vi "fitImageToWindow.vi"(8 "error in (no error)":errorcluster, 9 "Image Area Size":cluster{"Width":u32, "Height":u32}, 10 "ImageSize":cluster{"x":i32, "y":i32}, 11 "Snapper in":refnum<class "Snapper.lvclass">) -> (0 "error out":errorcluster, 2 "zoomInteger":cluster{dbl, dbl}, 3 "Snapper out":refnum<class "Snapper.lvclass">)   [LabVIEW 2009, in "Views.lvlib" / "Camera.lvlib" / "Snapper.lvclass"]
uses:
  Snapper.lvclass
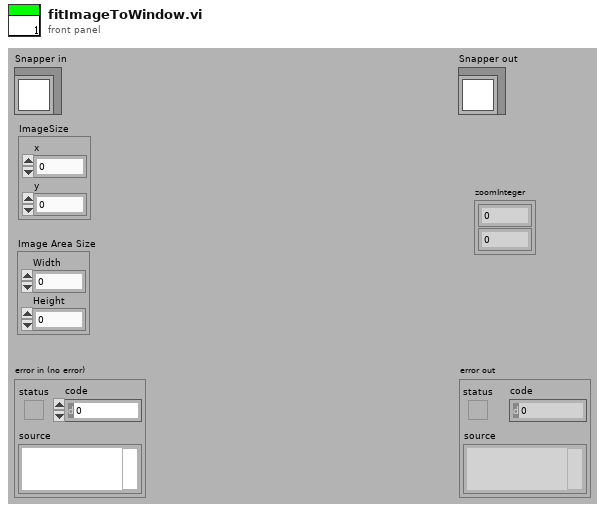
[diagram p1: front panel]
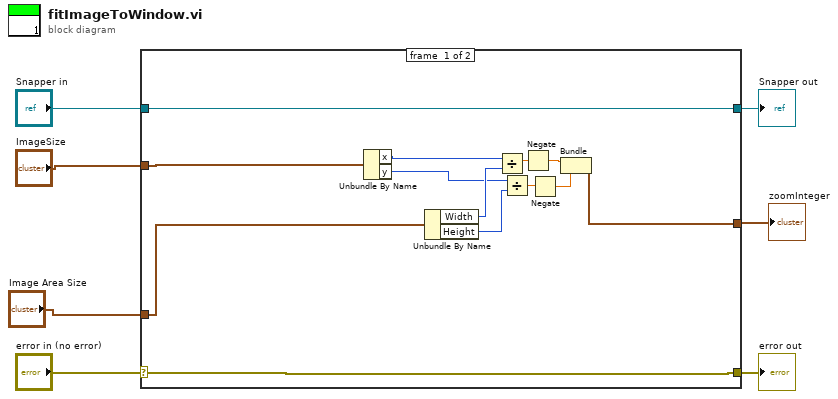
[diagram p0: block diagram]
diagram:
  n1 = case shown="No Error" "error in (no error)" {
    selector: "error in (no error)" -> [w8 w22]
    tunnel: [w8 w22] -> w6
    tunnel: [w20 w21] -> w4
    tunnel: "Snapper in" -> [w20 w21]
    tunnel: [w11 _] -> w3
    tunnel: "Image Area Size" -> [w10 _]
    tunnel: "ImageSize" -> [w9 _]
    frame #0 {
      n2 = Unbundle By Name(w9) -> ("x"=w19:i32, "y"=w17:i32)
      n3 = Unbundle By Name(w10) -> ("Width"=w18:u32, "Height"=w16:u32)
      n4 = Divide(x=w19, y=w18) -> (x/y=w15:dbl)
      n5 = Divide(x=w17, y=w16) -> (x/y=w14:dbl)
      n6 = Negate(x=w15) -> (-x=w13:dbl)
      n7 = Negate(x=w14) -> (-x=w12:dbl)
      n8 = Bundle(w13, w12) -> (w11:cluster{dbl, dbl})  [unwired: 1 in]
    }
    frame #1 {
    }
  }
  "error out" <- w6
  "Snapper out" <- w4
  "zoomInteger" <- w3
